vi "Begin.vi"() -> (0 "error out":errorcluster)   [LabVIEW 2012]
doc: "Called before other user functions, this VI is expected to open initial I/O refnums, load in file data, and do all program initialization. Notice that the <B>error out</B> terminal is simply used for data flow. Wiring it to other structures or subVIs ensures that this VI runs first."
uses:
  <vilib>/Rock Robotics/WPI/DriverStation/WPI_DriverStationRobotMode2.ctl
  <vilib>/Rock Robotics/SystemInterfaces/Typedef/FPGA_TypedefDigitalModule.ctl
  <vilib>/Rock Robotics/SystemInterfaces/DIO/FPGA_DIOPWMChannel.ctl
  <vilib>/Rock Robotics/SystemInterfaces/DIO/FPGA_DIOChannel.ctl
  <vilib>/Rock Robotics/WPI/Encoder/WPI_EncoderType.ctl
  <vilib>/Rock Robotics/WPI/Joystick/WPI_JoystickDeviceEnum.ctl
  <vilib>/Rock Robotics/SystemInterfaces/Typedef/FPGA_TypedefAnalogModule.ctl
  <vilib>/Rock Robotics/SystemInterfaces/AI/FPGA_AIChannel.ctl
  <vilib>/Rock Robotics/SystemInterfaces/DIO/FPGA_DIORelayChannel.ctl
  <vilib>/Rock Robotics/WPI/Relay/WPI_RelayDirection.ctl
  <vilib>/Rock Robotics/WPI/SafetyOutput/WPI_SafetyOutputConfigMenu.ctl
  Robot Global Data.vi
  <vilib>/Rock Robotics/WPI/MotorControl/WPI_MotorControlOpen Victor.vi
  <vilib>/Rock Robotics/WPI/MotorControl/WPI_MotorControlOpen Jaguar.vi
  <vilib>/Rock Robotics/WPI/Counter/WPI_CounterDigitalInputToDigitalSource.vi
  <vilib>/Rock Robotics/WPI/RobotDrive/WPI_RobotDriveOpen2MotorWithJaguar.vi
  <vilib>/Rock Robotics/WPI/RobotDrive/WPI_RobotDriveOpen4MotorWithJaguar.vi
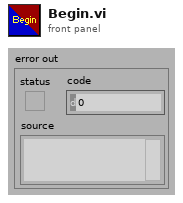
[diagram p1: front panel]
types:
  T1 = typedef "WPI_DriverStationRobotMode2.ctl" = enum16{"Autonomous Disabled", "Autonomous Enabled", "Teleop Disabled", "Teleop Enabled", "Timeout", "Finish", "Test Disabled", "Test Enabled"}
  T2 = typedef "FPGA_DIOChannel.ctl" = enum8{"DIO 1", "DIO 2", "DIO 3", "DIO 4", "DIO 5", "DIO 6", "DIO 7", "DIO 8", "DIO 9", "DIO 10", "DIO 11", "DIO 12", "DIO 13", "DIO 14", "Invalid"}
  T3 = typedef "FPGA_TypedefDigitalModule.ctl" = enum16{"Digital Module 1", "Digital Module 2"}
  T4 = typedef "WPI_DigitalInputDevRef.ctl" = cluster{"DevStatus":errorcluster, "DIO Channel":T2, "Digital Module":T3}
  T5 = typedef "WPI_SafetyOutputConfigMenu.ctl" = enum16{"Enable", "Disable"}
  T6 = typedef "FPGA_DIOPWMChannel.ctl" = enum8{"PWM 1", "PWM 2", "PWM 3", "PWM 4", "PWM 5", "PWM 6", "PWM 7", "PWM 8", "PWM 9", "PWM 10", "Invalid"}
  T7 = typedef "WPI_RobotDriveDevRef.ctl" = cluster{"DevStatus":errorcluster, "Motors[]":T8[], "Square Inputs":bool, "Max Output":dbl, "Isochronous":bool}
  T8 = typedef "WPI_MotorControlDeviceRef.ctl" = cluster{"DeviceStatus":errorcluster, "Type":enum16{"PWM", "CAN"}, "PWM":cluster{"Digital Module":T3, "PWM Channel":T6, "DeadBand":T9}, "CAN":cluster{"Device Number":u8, "Control Mode":T10, "Semaphore":T11, "Max Vout":dbl}, "Invert":bool, "TransformRef":T12, "InvTransformRef":T12}
  T9 = typedef "WPI_PWMDeadband.ctl" = cluster{"Name":string, "maxPositivePwm":i32, "minPositivePwm":i32, "centerPwm":i32, "maxNegativePwm":i32, "minNegativePwm":i32, "angularRange":u16}
  T10 = typedef "WPI_CANJaguar_ControlMode.ctl" = enum8{"Percent VBus", "Current", "Speed", "Position", "Voltage"}
  T11 = typedef "Semaphore RefNum" = refnum<k1>
  T12 = typedef "WPI_PWMTransform_ConPane.ctl" = refnum<vi>
  T13 = typedef "WPI_RelayDirection.ctl" = enum16{"Both directions", "Forward only", "Reverse only"}
  T14 = typedef "FPGA_DIORelayChannel.ctl" = enum8{"Relay 1", "Relay 2", "Relay 3", "Relay 4", "Relay 5", "Relay 6", "Relay 7", "Relay 8", "Invalid"}
  T15 = typedef "WPI_ServoDeviceRef.ctl" = cluster{"DeviceStatus":errorcluster, "Digital Module":T3, "PWM Channel":T6, "DeadBand":T9}
  T16 = typedef "WPI_RelayDevRef.ctl" = cluster{"DevStatus":errorcluster, "Relay Channel":T14, "Digital Module":T3, "Relay Direction":T13}
  T17 = typedef "WPI_JoystickDeviceEnum.ctl" = enum16{"USB 1", "USB 2", "USB 3", "USB 4", "Kinect 1", "Kinect 2"}
  T18 = typedef "WPI_JoystickDevRef.ctl" = cluster{"Device":T17}
  T19 = typedef "WPI_EncoderType.ctl" = enum16{"1x", "2x", "4x"}
  T20 = typedef "FPGA_CounterEncoderSourceConvertionLVSourceType.ctl" = cluster{"DevStatus":errorcluster, "AnalogTriggerMode?":bool, "DigitalMode":cluster{"Digital Module":T3, "DIO Channel":T21}, "AnalogTriggerMode":cluster{"AnalogTriggerIndex":T22, "OutputType":T23}}
  T21 = typedef "FPGA_DIODigitalSourceChannel.ctl" = enum8{"DIO 1", "DIO 2", "DIO 3", "DIO 4", "DIO 5", "DIO 6", "DIO 7", "DIO 8", "DIO 9", "DIO 10", "DIO 11", "DIO 12", "DIO 13", "DIO 14", "Disabled"}
  T22 = typedef "FPGA_AnalogTriggerIndex.ctl" = enum8{"Trig 0", "Trig 1", "Trig 2", "Trig 3", "Trig 4", "Trig 5", "Trig 6", "Trig 7", "Invalid"}
  T23 = typedef "FPGA_AnalogTriggerOutType.ctl" = enum16{"InWindow", "TriggerState", "Rising", "Falling"}
  T24 = typedef "WPI_EncoderDevRef.ctl" = cluster{"DevStatus":errorcluster, "EncoderIndex":T25, "CounterIndex":T26, "DistancePerCount":dbl, "Decoding Type":T19}
  T25 = typedef "FPGA_EncoderIdx.ctl" = enum8{"Enc 0", "Enc 1", "Enc 2", "Enc 3", "Invalid"}
  T26 = typedef "FPGA_CounterCtrSystemIndex.ctl" = enum8{"Ctr 0", "Ctr 1", "Ctr 2", "Ctr 3", "Ctr 4", "Ctr 5", "Ctr 6", "Ctr 7", "Invalid"}
  T27 = typedef "FPGA_AIChannel.ctl" = enum8{"AI 1", "AI 2", "AI 3", "AI 4", "AI 5", "AI 6", "AI 7", "AI 8", "Invalid"}
  T28 = typedef "FPGA_TypedefAnalogModule.ctl" = enum16{"Analog Module 1", "Analog Module 2"}
  T29 = typedef "WPI_AnalogChannelDevRef.ctl" = cluster{"DevStatus":errorcluster, "Analog Module":T28, "Analog Channel":T27}
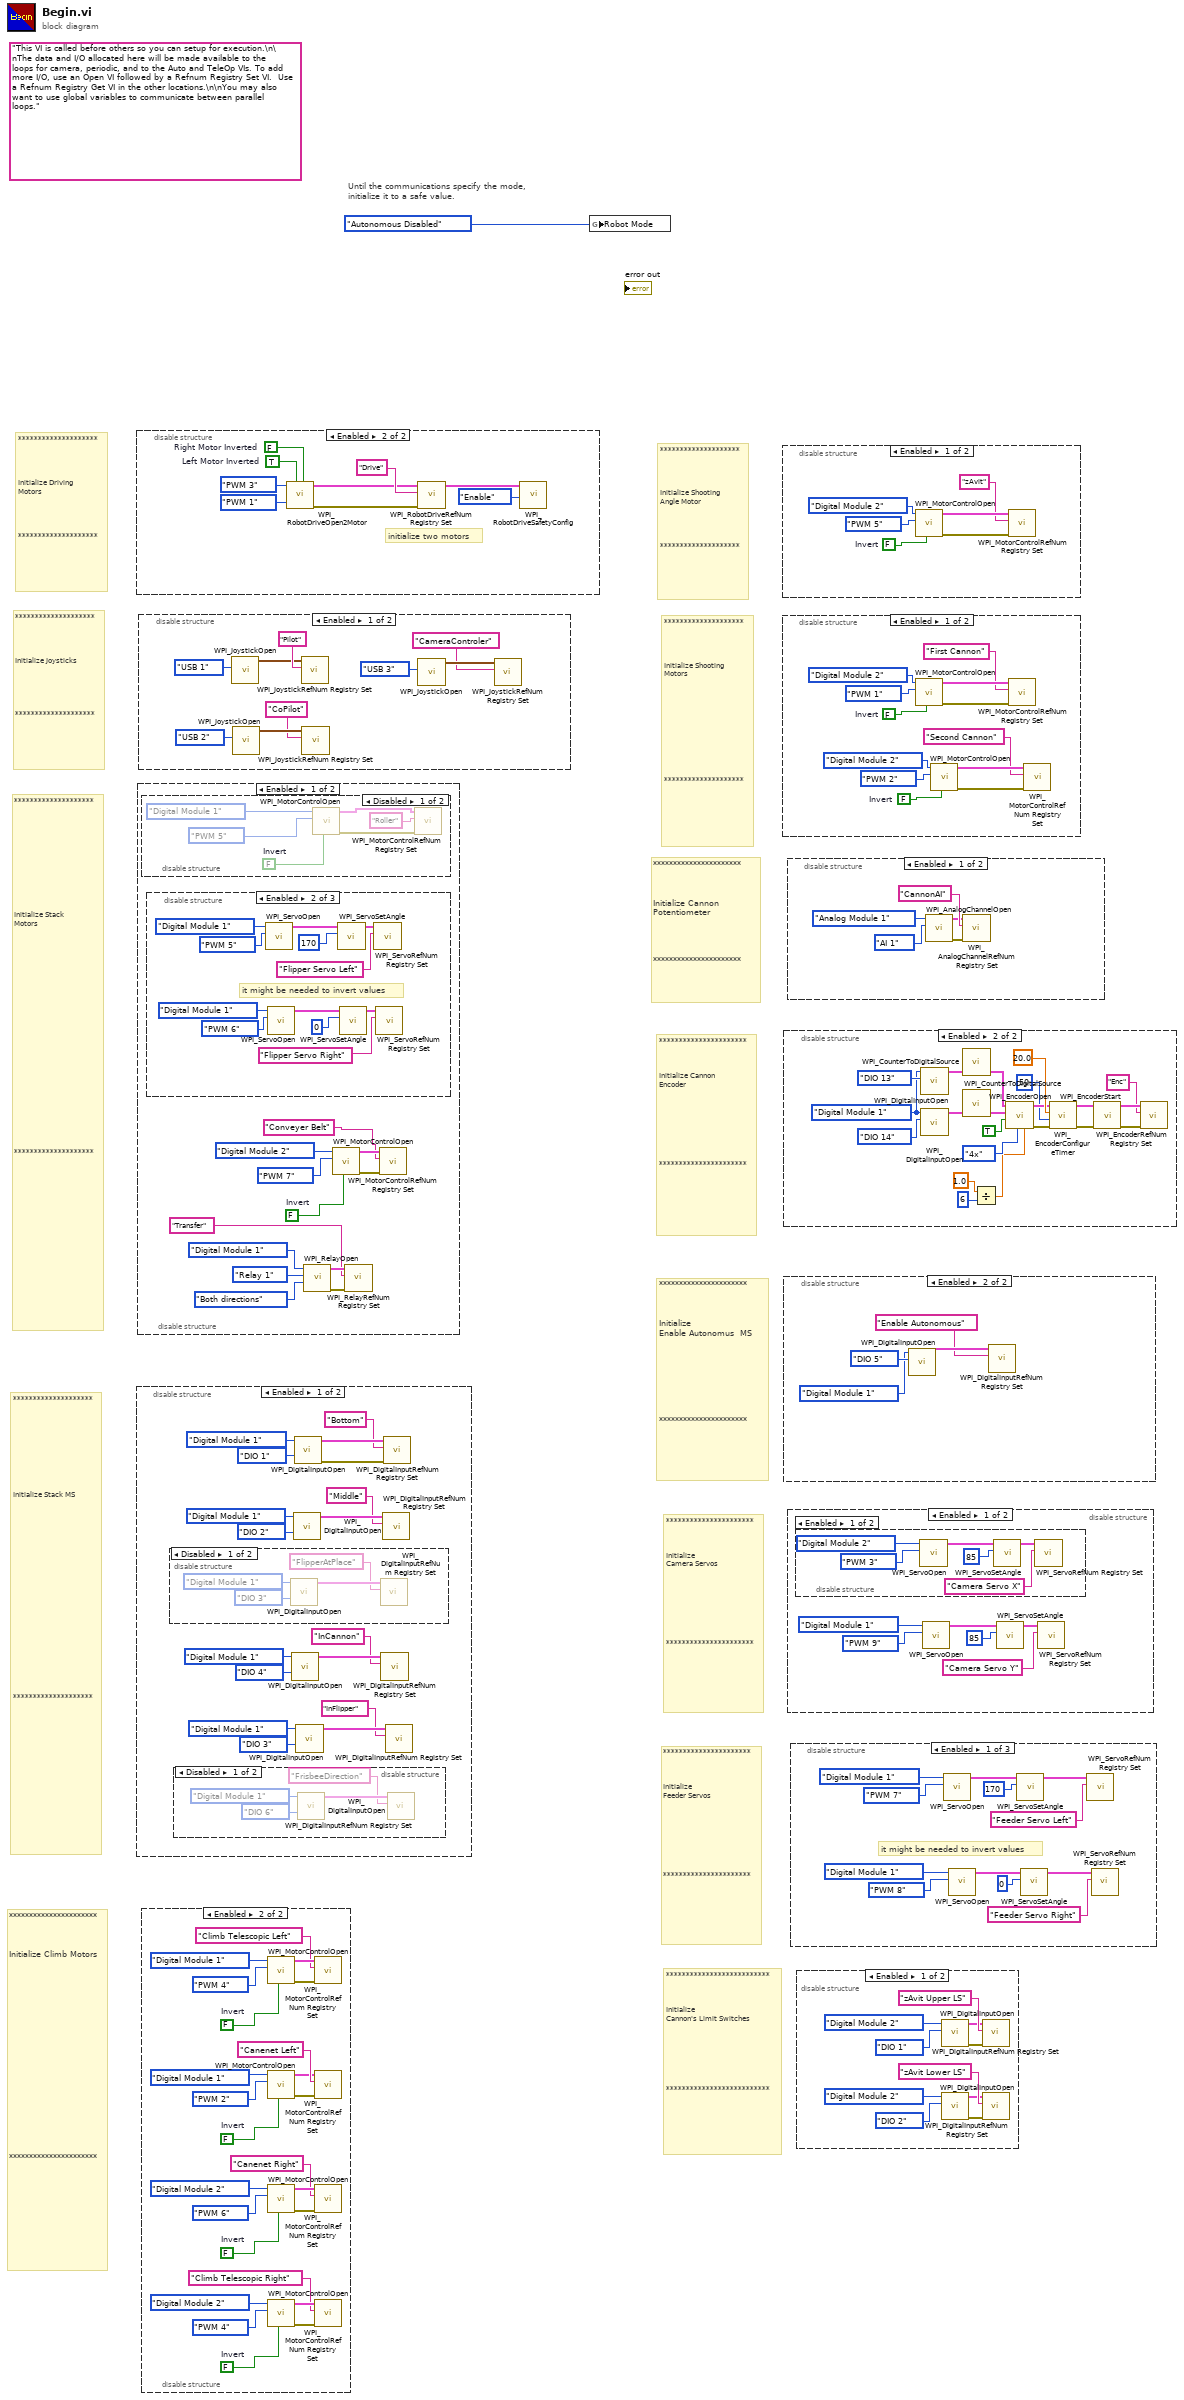
[diagram p0: block diagram]
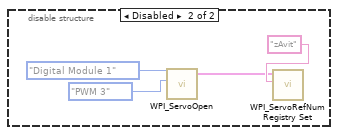
[diagram p9: hidden frame]
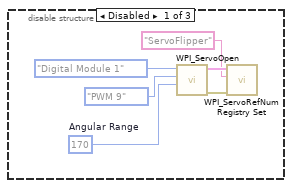
[diagram p18: hidden frame]
diagram:
  (unwired) "This VI is called before others so you can setup for execution.\n\nThe data and I/O allocated here will be made available to the loops for camera, periodic, and to the Auto and TeleOp VIs. To add more I/O, use an Open VI followed by a Refnum Registry Set VI.  Use a Refnum Registry Get VI in the other locations.\n\nYou may also want to use global variables to communicate between parallel loops."
  # "**************************\n\n\n\nInitialize\nCannon's Limit Switches\n\n\n\n\n\n\n\n**************************"
  # "**********************\n\n\n\nInitialize\nFeeder Servos\n\n\n\n\n\n\n\n\n**********************"
  # "**********************\n\n\n\nInitialize\nCamera Servos\n\n\n\n\n\n\n\n\n**********************"
  # "**********************\n\n\n\nInitialize Climb Motors          \n\n\n\n\n\n\n\n\n\n\n\n\n\n\n\n\n\n\n\n\n**********************"
  # "**********************\n\n\n\nInitialize\nEnable Autonomus  MS\n\n\n\n\n\n\n\n\n**********************"
  # "********************\n\n\n\n\nInitialize Shooting\nAngle Motor\n\n\n\n\n********************"
  # "**********************\n\n\n           \nInitialize Cannon Potentiometer\n\n\n\n\n**********************"
  # "**********************\n\n\n\nInitialize Cannon\nEncoder           \n\n\n\n\n\n\n\n\n**********************"
  # "********************\n\n\n\n\n\n\n\n\n\n\nInitialize Stack MS\n\n\n\n\n\n\n\n\n\n\n\n\n\n\n\n\n\n\n\n\n\n\n********************"
  # "********************\n\n\n\n\nInitialize Shooting\nMotors\n\n\n\n\n\n\n\n\n\n\n\n********************"
  # "********************\n\n\n\n\n\n\n\n\n\n\n\n\nInitialize Stack \nMotors\n\n\n\n\n\n\n\n\n\n\n\n\n\n\n\n\n\n\n\n\n\n\n\n\n\n********************"
  # "********************\n\n\n\n\nInitialize Driving\nMotors\n\n\n\n\n********************"
  # "********************\n\n\n\n\nInitialize Joysticks\n\n\n\n\n\n********************"
  # "Until the communications specify the mode,\ninitialize it to a safe value."
  n1 = disable-structure shown="Enabled" {
    frame Enabled {
      n2 = disable-structure shown="Disabled" {
        frame Disabled {
          n3 = call <vilib>:"WPI_DigitalInputOpen.vi"("DIO Channel"=FPGA_DIOChannel."DIO 3", "Digital Module (Module 1)"=FPGA_TypedefDigitalModule."Digital Module 1") -> ("DigitalInputDevRef"=w26:T4)  [unwired: 8 in, 1 out]
          n4 = call <vilib>:"WPI_DigitalInputRefNum Registry Set.vi"("refnum name"="FlipperAtPlace", "DigitalInputDevRef"=w26) -> ()  [unwired: 8 in, 2 out]
        }
        frame Enabled {
        }
      }
      n5 = disable-structure shown="Disabled" {
        frame Disabled {
          n6 = call <vilib>:"WPI_DigitalInputOpen.vi"("DIO Channel"=FPGA_DIOChannel."DIO 6", "Digital Module (Module 1)"=FPGA_TypedefDigitalModule."Digital Module 1") -> ("DigitalInputDevRef"=w20:T4)  [unwired: 8 in, 1 out]
          n7 = call <vilib>:"WPI_DigitalInputRefNum Registry Set.vi"("refnum name"="FrisbeeDirection", "DigitalInputDevRef"=w20) -> ()  [unwired: 8 in, 2 out]
        }
        frame Enabled {
        }
      }
      n8 = call <vilib>:"WPI_DigitalInputOpen.vi"("DIO Channel"=FPGA_DIOChannel."DIO 4", "Digital Module (Module 1)"=FPGA_TypedefDigitalModule."Digital Module 1") -> ("DigitalInputDevRef"=w11:T4)  [unwired: 8 in, 1 out]
      n9 = call <vilib>:"WPI_DigitalInputOpen.vi"("DIO Channel"=FPGA_DIOChannel."DIO 2", "Digital Module (Module 1)"=FPGA_TypedefDigitalModule."Digital Module 1") -> ("DigitalInputDevRef"=w14:T4)  [unwired: 8 in, 1 out]
      n10 = call <vilib>:"WPI_DigitalInputOpen.vi"("DIO Channel"=FPGA_DIOChannel."DIO 1", "Digital Module (Module 1)"=FPGA_TypedefDigitalModule."Digital Module 1") -> ("error out"=w17:errorcluster, "DigitalInputDevRef"=w18:T4)  [unwired: 8 in]
      n11 = call <vilib>:"WPI_DigitalInputOpen.vi"("DIO Channel"=FPGA_DIOChannel."DIO 3", "Digital Module (Module 1)"=FPGA_TypedefDigitalModule."Digital Module 1") -> ("DigitalInputDevRef"=w8:T4)  [unwired: 8 in, 1 out]
      n12 = call <vilib>:"WPI_DigitalInputRefNum Registry Set.vi"("refnum name"="InCannon", "DigitalInputDevRef"=w11) -> ()  [unwired: 8 in, 2 out]
      n13 = call <vilib>:"WPI_DigitalInputRefNum Registry Set.vi"("refnum name"="Middle", "DigitalInputDevRef"=w14) -> ()  [unwired: 8 in, 2 out]
      n14 = call <vilib>:"WPI_DigitalInputRefNum Registry Set.vi"("error in (no error)"=w17, "refnum name"="Bottom", "DigitalInputDevRef"=w18) -> ()  [unwired: 7 in, 2 out]
      n15 = call <vilib>:"WPI_DigitalInputRefNum Registry Set.vi"("refnum name"="InFlipper", "DigitalInputDevRef"=w8) -> ()  [unwired: 8 in, 2 out]
    }
    frame Disabled {
    }
  }
  n16 = disable-structure shown="Enabled" {
    frame Disabled {
      w27 = FPGA_DIOPWMChannel."PWM 4"  # Front Right Motor
      w28 = FPGA_DIOPWMChannel."PWM 3"  # Front Left Motor
      w29 = FPGA_DIOPWMChannel."PWM 2"  # Rear Right Motor
      w30 = FPGA_DIOPWMChannel."PWM 1"  # Rear Left Motor
      w31 = FALSE  # Front Right Motor Inverted
      w32 = FALSE  # Front Left Motor Inverted
      w33 = FALSE  # Rear Right Motor Inverted
      w34 = FALSE  # Rear Left Motor Inverted
      # "initialize two motors"
      n17 = call-poly <vilib>:"WPI_RobotDriveOpen4Motor.vi"("Rear Left Motor"=w30, "Rear Left Motor Inverted"=w34, "Rear Right Motor Inverted"=w33, "Rear Right Motor"=w29, "Front Left Motor"=w28, "Front Right Motor"=w27, "Front Left Motor Inverted"=w32, "Front Right Motor Inverted"=w31) -> ("RobotDriveDevRef"=w36:T7, "error out"=w35:errorcluster)  [unwired: 6 in]
      n18 = call <vilib>:"WPI_RobotDriveRefNum Registry Set.vi"("error in (no error)"=w35, "refnum name"="Drive", "RobotDriveDevRef"=w36) -> ("RobotDriveDevRef"=w38:T7)  [unwired: 8 out]
      n19 = call <vilib>:"WPI_RobotDriveSafetyConfig.vi"("mode"=WPI_SafetyOutputConfigMenu."Enable", "RobotDriveDevRef"=w38) -> ()  [unwired: 8 in, 2 out]
    }
    frame Enabled {
      w40 = FALSE  # Right Motor Inverted
      w41 = TRUE  # Left Motor Inverted
      # "initialize two motors"
      n20 = call-poly <vilib>:"WPI_RobotDriveOpen2Motor.vi"("Right Motor Inverted"=w40, "Left Motor Inverted"=w41, "Right Motor"=FPGA_DIOPWMChannel."PWM 1", "Left Motor"=FPGA_DIOPWMChannel."PWM 3") -> ("error out"=w44:errorcluster, "RobotDriveDevRef"=w45:T7)  [unwired: 6 in]
      n21 = call <vilib>:"WPI_RobotDriveRefNum Registry Set.vi"("error in (no error)"=w44, "refnum name"="Drive", "RobotDriveDevRef"=w45) -> ("RobotDriveDevRef"=w47:T7)  [unwired: 8 out]
      n22 = call <vilib>:"WPI_RobotDriveSafetyConfig.vi"("mode"=WPI_SafetyOutputConfigMenu."Enable", "RobotDriveDevRef"=w47) -> ()  [unwired: 8 in, 2 out]
    }
  }
  n23 = disable-structure shown="Enabled" {
    frame Enabled {
      w51 = FALSE  # Invert
      n24 = disable-structure shown="Disabled" {
        frame Disabled {
          w62 = FALSE  # Invert
          n25 = call-poly <vilib>:"WPI_MotorControlOpen.vi"("Invert"=w62, "PWM Channel"=FPGA_DIOPWMChannel."PWM 5", "Digital Module (Module 1)"=FPGA_TypedefDigitalModule."Digital Module 1") -> ("error out"=w61:errorcluster, "MotorControlDeviceRef"=w66:T8)  [unwired: 7 in]
          n26 = call <vilib>:"WPI_MotorControlRefNum Registry Set.vi"("error in (no error)"=w61, "refnum name"="Roller", "MotorControlDevRef"=w66) -> ()  [unwired: 7 in, 2 out]
        }
        frame Enabled {
        }
      }
      n27 = disable-structure shown="Enabled" {
        frame Disabled {
          w69 = u16 170  # Angular Range
          n28 = call <vilib>:"WPI_ServoOpen.vi"("Angular Range"=w69, "PWM Channel"=FPGA_DIOPWMChannel."PWM 9", "Digital Module (Module 1)"=FPGA_TypedefDigitalModule."Digital Module 1") -> ("error out"=w68:errorcluster, "ServoDeviceRef"=w72:T15)  [unwired: 7 in]
          n29 = call <vilib>:"WPI_ServoRefNum Registry Set.vi"("error in (no error)"=w68, "refnum name"="ServoFlipper", "ServoDeviceRef"=w72) -> ()  [unwired: 7 in, 2 out]
        }
        frame Enabled {
          # "it might be needed to invert values"
          n30 = call <vilib>:"WPI_ServoOpen.vi"("PWM Channel"=FPGA_DIOPWMChannel."PWM 5", "Digital Module (Module 1)"=FPGA_TypedefDigitalModule."Digital Module 1") -> ("ServoDeviceRef"=w84:T15)  [unwired: 8 in, 1 out]
          n31 = call <vilib>:"WPI_ServoOpen.vi"("PWM Channel"=FPGA_DIOPWMChannel."PWM 6", "Digital Module (Module 1)"=FPGA_TypedefDigitalModule."Digital Module 1") -> ("ServoDeviceRef"=w74:T15)  [unwired: 8 in, 1 out]
          n32 = call <vilib>:"WPI_ServoSetAngle.vi"("Angle"=170, "ServoDeviceRef"=w84) -> ("ServoDeviceRef"=w80:T15)  [unwired: 8 in, 1 out]
          n33 = call <vilib>:"WPI_ServoSetAngle.vi"("Angle"=0, "ServoDeviceRef"=w74) -> ("ServoDeviceRef"=w77:T15)  [unwired: 8 in, 1 out]
          n34 = call <vilib>:"WPI_ServoRefNum Registry Set.vi"("refnum name"="Flipper Servo Left", "ServoDeviceRef"=w80) -> ()  [unwired: 8 in, 2 out]
          n35 = call <vilib>:"WPI_ServoRefNum Registry Set.vi"("refnum name"="Flipper Servo Right", "ServoDeviceRef"=w77) -> ()  [unwired: 8 in, 2 out]
        }
        frame Disabled {
        }
      }
      n36 = call <vilib>:"WPI_RelayOpen.vi"("Relay Direction"=WPI_RelayDirection."Both directions", "Relay Channel"=FPGA_DIORelayChannel."Relay 1", "Digital Module (Module 1)"=FPGA_TypedefDigitalModule."Digital Module 1") -> ("error out"=w57:errorcluster, "RelayDevRef"=w56:T16)  [unwired: 7 in]
      n37 = call-poly <vilib>:"WPI_MotorControlOpen.vi"("Invert"=w51, "PWM Channel"=FPGA_DIOPWMChannel."PWM 7", "Digital Module (Module 1)"=FPGA_TypedefDigitalModule."Digital Module 2") -> ("error out"=w50:errorcluster, "MotorControlDeviceRef"=w54:T8)  [unwired: 7 in]
      n38 = call <vilib>:"WPI_RelayRefNum Registry Set.vi"("error in (no error)"=w57, "refnum name"="Transfer", "RelayDevRef"=w56) -> ()  [unwired: 7 in, 2 out]
      n39 = call <vilib>:"WPI_MotorControlRefNum Registry Set.vi"("error in (no error)"=w50, "refnum name"="Conveyer Belt", "MotorControlDevRef"=w54) -> ()  [unwired: 7 in, 2 out]
    }
    frame Disabled {
    }
  }
  n40 = disable-structure shown="Enabled" {
    frame Enabled {
      n41 = call <vilib>:"WPI_JoystickOpen.vi"("JoystickDevice"=WPI_JoystickDeviceEnum."USB 1") -> ("JoystickDevRef"=w92:T18)  [unwired: 10 in]
      n42 = call <vilib>:"WPI_JoystickOpen.vi"("JoystickDevice"=WPI_JoystickDeviceEnum."USB 2") -> ("JoystickDevRef"=w89:T18)  [unwired: 10 in]
      n43 = call <vilib>:"WPI_JoystickRefNum Registry Set.vi"("refnum name"="Pilot", "JoystickDevRef"=w92) -> ()  [unwired: 8 in, 2 out]
      n44 = call <vilib>:"WPI_JoystickRefNum Registry Set.vi"("refnum name"="CoPilot", "JoystickDevRef"=w89) -> ()  [unwired: 8 in, 2 out]
      n45 = call <vilib>:"WPI_JoystickOpen.vi"("JoystickDevice"=WPI_JoystickDeviceEnum."USB 3") -> ("JoystickDevRef"=w86:T18)  [unwired: 10 in]
      n46 = call <vilib>:"WPI_JoystickRefNum Registry Set.vi"("refnum name"="CameraControler", "JoystickDevRef"=w86) -> ()  [unwired: 8 in, 2 out]
    }
    frame Disabled {
    }
  }
  n47 = disable-structure shown="Enabled" {
    frame Disabled {
    }
    frame Enabled {
      w97 = FALSE  # Invert
      w104 = FALSE  # Invert
      w110 = FALSE  # Invert
      w113 = FALSE  # Invert
      n48 = call-poly <vilib>:"WPI_MotorControlOpen.vi"("Invert"=w97, "PWM Channel"=FPGA_DIOPWMChannel."PWM 4", "Digital Module (Module 1)"=FPGA_TypedefDigitalModule."Digital Module 1") -> ("error out"=w96:errorcluster, "MotorControlDeviceRef"=w100:T8)  [unwired: 7 in]
      n49 = call-poly <vilib>:"WPI_MotorControlOpen.vi"("Invert"=w110, "PWM Channel"=FPGA_DIOPWMChannel."PWM 2", "Digital Module (Module 1)"=FPGA_TypedefDigitalModule."Digital Module 1") -> ("error out"=w111:errorcluster, "MotorControlDeviceRef"=w106:T8)  [unwired: 7 in]
      n50 = call-poly <vilib>:"WPI_MotorControlOpen.vi"("Invert"=w113, "PWM Channel"=FPGA_DIOPWMChannel."PWM 6", "Digital Module (Module 1)"=FPGA_TypedefDigitalModule."Digital Module 2") -> ("error out"=w112:errorcluster, "MotorControlDeviceRef"=w117:T8)  [unwired: 7 in]
      n51 = call-poly <vilib>:"WPI_MotorControlOpen.vi"("Invert"=w104, "PWM Channel"=FPGA_DIOPWMChannel."PWM 4", "Digital Module (Module 1)"=FPGA_TypedefDigitalModule."Digital Module 2") -> ("error out"=w105:errorcluster, "MotorControlDeviceRef"=w101:T8)  [unwired: 7 in]
      n52 = call <vilib>:"WPI_MotorControlRefNum Registry Set.vi"("error in (no error)"=w96, "refnum name"="Climb Telescopic Left", "MotorControlDevRef"=w100) -> ()  [unwired: 7 in, 2 out]
      n53 = call <vilib>:"WPI_MotorControlRefNum Registry Set.vi"("error in (no error)"=w111, "refnum name"="Canenet Left", "MotorControlDevRef"=w106) -> ()  [unwired: 7 in, 2 out]
      n54 = call <vilib>:"WPI_MotorControlRefNum Registry Set.vi"("error in (no error)"=w112, "refnum name"="Canenet Right", "MotorControlDevRef"=w117) -> ()  [unwired: 7 in, 2 out]
      n55 = call <vilib>:"WPI_MotorControlRefNum Registry Set.vi"("error in (no error)"=w105, "refnum name"="Climb Telescopic Right", "MotorControlDevRef"=w101) -> ()  [unwired: 7 in, 2 out]
    }
  }
  n56 = global write "Robot Global Data.vi" "Robot Mode"(WPI_DriverStationRobotMode2."Autonomous Disabled" ("Robot Mode")) -> ()
  n57 = disable-structure shown="Enabled" {
    frame Enabled {
      w119 = FALSE  # Invert
      n58 = call-poly <vilib>:"WPI_MotorControlOpen.vi"("Invert"=w119, "PWM Channel"=FPGA_DIOPWMChannel."PWM 5", "Digital Module (Module 1)"=FPGA_TypedefDigitalModule."Digital Module 2") -> ("error out"=w118:errorcluster, "MotorControlDeviceRef"=w123:T8)  [unwired: 7 in]
      n59 = call <vilib>:"WPI_MotorControlRefNum Registry Set.vi"("error in (no error)"=w118, "refnum name"="zAvit", "MotorControlDevRef"=w123) -> ()  [unwired: 7 in, 2 out]
    }
    frame Disabled {
      n60 = call <vilib>:"WPI_ServoOpen.vi"("PWM Channel"=FPGA_DIOPWMChannel."PWM 3", "Digital Module (Module 1)"=FPGA_TypedefDigitalModule."Digital Module 1") -> ("ServoDeviceRef"=w124:T15)  [unwired: 8 in, 1 out]
      n61 = call <vilib>:"WPI_ServoRefNum Registry Set.vi"("refnum name"="zAvit", "ServoDeviceRef"=w124) -> ()  [unwired: 8 in, 2 out]
    }
  }
  n62 = disable-structure shown="Enabled" {
    frame Enabled {
      w129 = FALSE  # Invert
      w135 = FALSE  # Invert
      n63 = call-poly <vilib>:"WPI_MotorControlOpen.vi"("Invert"=w135, "PWM Channel"=FPGA_DIOPWMChannel."PWM 1", "Digital Module (Module 1)"=FPGA_TypedefDigitalModule."Digital Module 2") -> ("error out"=w134:errorcluster, "MotorControlDeviceRef"=w139:T8)  [unwired: 7 in]
      n64 = call-poly <vilib>:"WPI_MotorControlOpen.vi"("Invert"=w129, "PWM Channel"=FPGA_DIOPWMChannel."PWM 2", "Digital Module (Module 1)"=FPGA_TypedefDigitalModule."Digital Module 2") -> ("error out"=w128:errorcluster, "MotorControlDeviceRef"=w133:T8)  [unwired: 7 in]
      n65 = call <vilib>:"WPI_MotorControlRefNum Registry Set.vi"("error in (no error)"=w134, "refnum name"="First Cannon", "MotorControlDevRef"=w139) -> ()  [unwired: 7 in, 2 out]
      n66 = call <vilib>:"WPI_MotorControlRefNum Registry Set.vi"("error in (no error)"=w128, "refnum name"="Second Cannon", "MotorControlDevRef"=w133) -> ()  [unwired: 7 in, 2 out]
    }
    frame Disabled {
    }
  }
  n67 = disable-structure shown="Enabled" {
    frame Disabled {
    }
    frame Enabled {
      w143 = FPGA_TypedefDigitalModule."Digital Module 1" ("DIO Module")
      n68 = call <vilib>:"WPI_DigitalInputOpen.vi"("DIO Channel"=FPGA_DIOChannel."DIO 13" ("A Channel"), "Digital Module (Module 1)"=w143) -> ("DigitalInputDevRef"=w152:T4)  [unwired: 1 in, 8 out]
      n69 = call <vilib>:"WPI_DigitalInputOpen.vi"("DIO Channel"=FPGA_DIOChannel."DIO 14" ("B Channel"), "Digital Module (Module 1)"=w143) -> ("DigitalInputDevRef"=w153:T4)  [unwired: 1 in, 8 out]
      n70 = call-poly <vilib>:"WPI_CounterToDigitalSource.vi"("DigitalInputDevRef"=w152) -> ("Digital Source"=w151:T20)  [unwired: 6 out]
      n71 = call-poly <vilib>:"WPI_CounterToDigitalSource.vi"("DigitalInputDevRef"=w153) -> ("Digital Source"=w154:T20)  [unwired: 6 out]
      n72 = Divide(x=1.0 ("DistancePerCount"), y=6) -> (x/y=w140:dbl)
      n73 = call <vilib>:"WPI_EncoderOpen.vi"("DistancePerCount"=w140, "Decoding Type"=WPI_EncoderType."4x", "Invert Direction (False)"=TRUE ("Invert Direction"), "BSource"=w154, "ASource"=w151) -> ("error out"=w158:errorcluster, "EncoderDevRef"=w145:T24)  [unwired: 3 in, 2 out]
      n74 = call <vilib>:"WPI_EncoderConfigureTimer.vi"("error in (no error)"=w158, "Number Samples to Average"=u8 50, "Minimum Rate"=20.0, "EncoderDevRef"=w145) -> ("error out"=w159:errorcluster, "EncoderDevRef"=w146:T24)  [unwired: 6 out]
      n75 = call <vilib>:"WPI_EncoderStart.vi"("error in (no error)"=w159, "EncoderDevRef"=w146) -> ("error out"=w160:errorcluster, "EncoderDevRef"=w157:T24)  [unwired: 8 out]
      n76 = call <vilib>:"WPI_EncoderRefNum Registry Set.vi"("error in (no error)"=w160, "refnum name"="Enc", "EncoderDevRef"=w157) -> ()  [unwired: 9 out]
    }
  }
  n77 = disable-structure shown="Enabled" {
    frame Disabled {
    }
    frame Enabled {
      n78 = call <vilib>:"WPI_DigitalInputOpen.vi"("DIO Channel"=FPGA_DIOChannel."DIO 5" ("A Channel"), "Digital Module (Module 1)"=FPGA_TypedefDigitalModule."Digital Module 1" ("DIO Module")) -> ("DigitalInputDevRef"=w162:T4)  [unwired: 1 in, 8 out]
      n79 = call <vilib>:"WPI_DigitalInputRefNum Registry Set.vi"("refnum name"="Enable Autonomous", "DigitalInputDevRef"=w162) -> ()  [unwired: 8 in, 2 out]
    }
  }
  n80 = disable-structure shown="Enabled" {
    frame Enabled {
      n81 = call <vilib>:"WPI_AnalogChannelOpen.vi"("Analog Channel"=FPGA_AIChannel."AI 1", "Analog Module (Module 1)"=FPGA_TypedefAnalogModule."Analog Module 1") -> ("error out"=w166:errorcluster, "AIDeviceRef"=w165:T29)  [unwired: 8 in]
      n82 = call <vilib>:"WPI_AnalogChannelRefNum Registry Set.vi"("error in (no error)"=w166, "refnum name"="CannonAI", "AIDeviceRef"=w165) -> ()  [unwired: 7 in, 2 out]
    }
    frame Disabled {
    }
  }
  n83 = disable-structure shown="Enabled" {
    frame Enabled {
      n84 = disable-structure shown="Enabled" {
        frame Enabled {
          n85 = call <vilib>:"WPI_ServoOpen.vi"("PWM Channel"=FPGA_DIOPWMChannel."PWM 3", "Digital Module (Module 1)"=FPGA_TypedefDigitalModule."Digital Module 2") -> ("ServoDeviceRef"=w178:T15)  [unwired: 8 in, 1 out]
          n86 = call <vilib>:"WPI_ServoSetAngle.vi"("Angle"=85, "ServoDeviceRef"=w178) -> ("ServoDeviceRef"=w177:T15)  [unwired: 8 in, 1 out]
          n87 = call <vilib>:"WPI_ServoRefNum Registry Set.vi"("refnum name"="Camera Servo X", "ServoDeviceRef"=w177) -> ()  [unwired: 8 in, 2 out]
        }
        frame Disabled {
        }
      }
      n88 = call <vilib>:"WPI_ServoOpen.vi"("PWM Channel"=FPGA_DIOPWMChannel."PWM 9", "Digital Module (Module 1)"=FPGA_TypedefDigitalModule."Digital Module 1") -> ("ServoDeviceRef"=w173:T15)  [unwired: 8 in, 1 out]
      n89 = call <vilib>:"WPI_ServoSetAngle.vi"("Angle"=85, "ServoDeviceRef"=w173) -> ("ServoDeviceRef"=w174:T15)  [unwired: 8 in, 1 out]
      n90 = call <vilib>:"WPI_ServoRefNum Registry Set.vi"("refnum name"="Camera Servo Y", "ServoDeviceRef"=w174) -> ()  [unwired: 8 in, 2 out]
    }
    frame Disabled {
    }
  }
  n91 = disable-structure shown="Enabled" {
    frame Enabled {
      # "it might be needed to invert values"
      n92 = call <vilib>:"WPI_ServoOpen.vi"("PWM Channel"=FPGA_DIOPWMChannel."PWM 7", "Digital Module (Module 1)"=FPGA_TypedefDigitalModule."Digital Module 1") -> ("ServoDeviceRef"=w190:T15)  [unwired: 8 in, 1 out]
      n93 = call <vilib>:"WPI_ServoOpen.vi"("PWM Channel"=FPGA_DIOPWMChannel."PWM 8", "Digital Module (Module 1)"=FPGA_TypedefDigitalModule."Digital Module 1") -> ("ServoDeviceRef"=w189:T15)  [unwired: 8 in, 1 out]
      n94 = call <vilib>:"WPI_ServoSetAngle.vi"("Angle"=170, "ServoDeviceRef"=w190) -> ("ServoDeviceRef"=w185:T15)  [unwired: 8 in, 1 out]
      n95 = call <vilib>:"WPI_ServoSetAngle.vi"("Angle"=0, "ServoDeviceRef"=w189) -> ("ServoDeviceRef"=w184:T15)  [unwired: 8 in, 1 out]
      n96 = call <vilib>:"WPI_ServoRefNum Registry Set.vi"("refnum name"="Feeder Servo Left", "ServoDeviceRef"=w185) -> ()  [unwired: 8 in, 2 out]
      n97 = call <vilib>:"WPI_ServoRefNum Registry Set.vi"("refnum name"="Feeder Servo Right", "ServoDeviceRef"=w184) -> ()  [unwired: 8 in, 2 out]
    }
    frame Disabled {
    }
    frame Disabled {
    }
  }
  n98 = disable-structure shown="Enabled" {
    frame Enabled {
      n99 = call <vilib>:"WPI_DigitalInputOpen.vi"("DIO Channel"=FPGA_DIOChannel."DIO 1", "Digital Module (Module 1)"=FPGA_TypedefDigitalModule."Digital Module 2") -> ("error out"=w199:errorcluster, "DigitalInputDevRef"=w200:T4)  [unwired: 8 in]
      n100 = call <vilib>:"WPI_DigitalInputOpen.vi"("DIO Channel"=FPGA_DIOChannel."DIO 2", "Digital Module (Module 1)"=FPGA_TypedefDigitalModule."Digital Module 2") -> ("error out"=w198:errorcluster, "DigitalInputDevRef"=w201:T4)  [unwired: 8 in]
      n101 = call <vilib>:"WPI_DigitalInputRefNum Registry Set.vi"("error in (no error)"=w199, "refnum name"="zAvit Upper LS", "DigitalInputDevRef"=w200) -> ()  [unwired: 7 in, 2 out]
      n102 = call <vilib>:"WPI_DigitalInputRefNum Registry Set.vi"("error in (no error)"=w198, "refnum name"="zAvit Lower LS", "DigitalInputDevRef"=w201) -> ()  [unwired: 7 in, 2 out]
    }
    frame Disabled {
    }
  }
